vi "Autonomous Independent.vi"() -> ()   [LabVIEW 2012]
doc: "This VI is called when autonomous begins, and will automatically be terminated when autonomous ends. You can carry out timed or sensor driven robot movement independently without needing to return to the caller."
uses:
  Robot Global Data.vi
  <vilib>/Rock Robotics/WPI/RobotDrive/WPI_RobotDriveGetSetRefNum.vi
  <vilib>/Rock Robotics/WPI/Joystick/WPI_JoystickGetSetRefNum.vi
panel:
  out "Current Movement, for debugging":T1 {"Y Joystick Value" scale=1.0..-1.0; "X Joystick Value" scale=-1.0..1.0}
  in  "Array of robot movements":T2(array[cluster]) {"Y Joystick Value" scale=1.0..-1.0; "X Joystick Value" scale=-1.0..1.0}
  # "Be sure to right-click and choose Data Operations>>Make Current Value default if you want to save the array values with the VI"
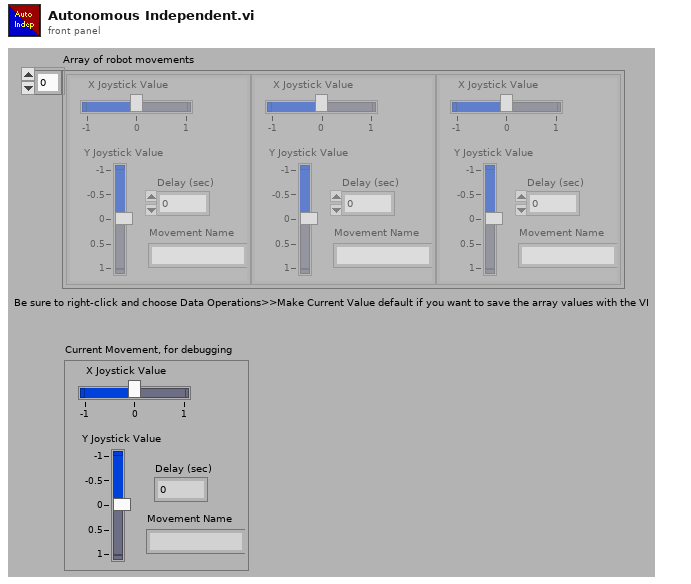
[diagram p1: front panel]
types:
  T1 = cluster{"X Joystick Value":dbl, "Y Joystick Value":dbl, "Delay (sec)":dbl, "Movement Name":string}
  T2 = cluster{"X Joystick Value":dbl, "Y Joystick Value":dbl, "Delay (sec)":dbl, "Movement Name":string}[]
  T3 = typedef "WPI_JoystickDevRef.ctl" = cluster{"Device":T4}
  T4 = typedef "WPI_JoystickDeviceEnum.ctl" = enum16{"USB 1", "USB 2", "USB 3", "USB 4", "Kinect 1", "Kinect 2"}
  T5 = cluster{"axis 1 (x)":dbl, "axis 2 (y)":dbl, "axis 3 (throttle)":dbl, "axis 4":dbl, "axis 5":dbl, "axis 6":dbl}
  T6 = typedef "WPI_RobotDriveDevRef.ctl" = cluster{"DevStatus":errorcluster, "Motors[]":T7[], "Square Inputs":bool, "Max Output":dbl, "Isochronous":bool}
  T7 = typedef "WPI_MotorControlDeviceRef.ctl" = cluster{"DeviceStatus":errorcluster, "Type":enum16{"PWM", "CAN"}, "PWM":cluster{"Digital Module":T8, "PWM Channel":T9, "DeadBand":T10}, "CAN":cluster{"Device Number":u8, "Control Mode":T11, "Semaphore":T12, "Max Vout":dbl}, "Invert":bool, "TransformRef":T13, "InvTransformRef":T13}
  T8 = typedef "FPGA_TypedefDigitalModule.ctl" = enum16{"Digital Module 1", "Digital Module 2"}
  T9 = typedef "FPGA_DIOPWMChannel.ctl" = enum8{"PWM 1", "PWM 2", "PWM 3", "PWM 4", "PWM 5", "PWM 6", "PWM 7", "PWM 8", "PWM 9", "PWM 10", "Invalid"}
  T10 = typedef "WPI_PWMDeadband.ctl" = cluster{"Name":string, "maxPositivePwm":i32, "minPositivePwm":i32, "centerPwm":i32, "maxNegativePwm":i32, "minNegativePwm":i32, "angularRange":u16}
  T11 = typedef "WPI_CANJaguar_ControlMode.ctl" = enum8{"Percent VBus", "Current", "Speed", "Position", "Voltage"}
  T12 = typedef "Semaphore RefNum" = refnum<k1>
  T13 = typedef "WPI_PWMTransform_ConPane.ctl" = refnum<vi>
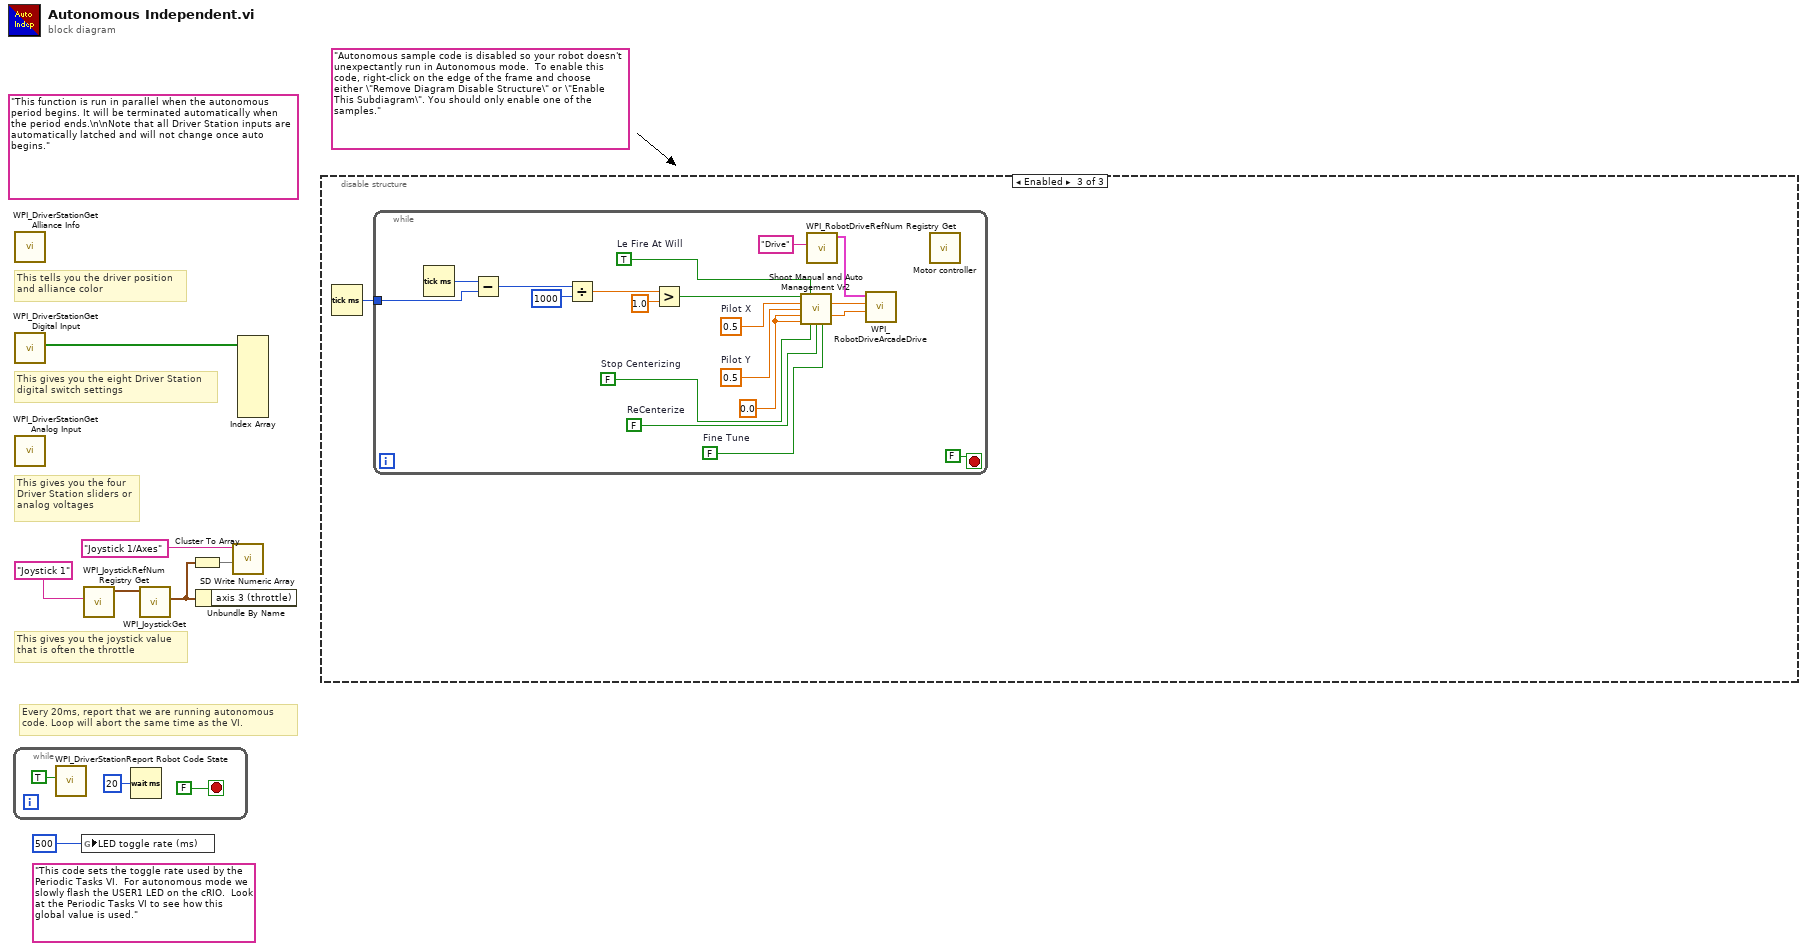
[diagram p0: block diagram]
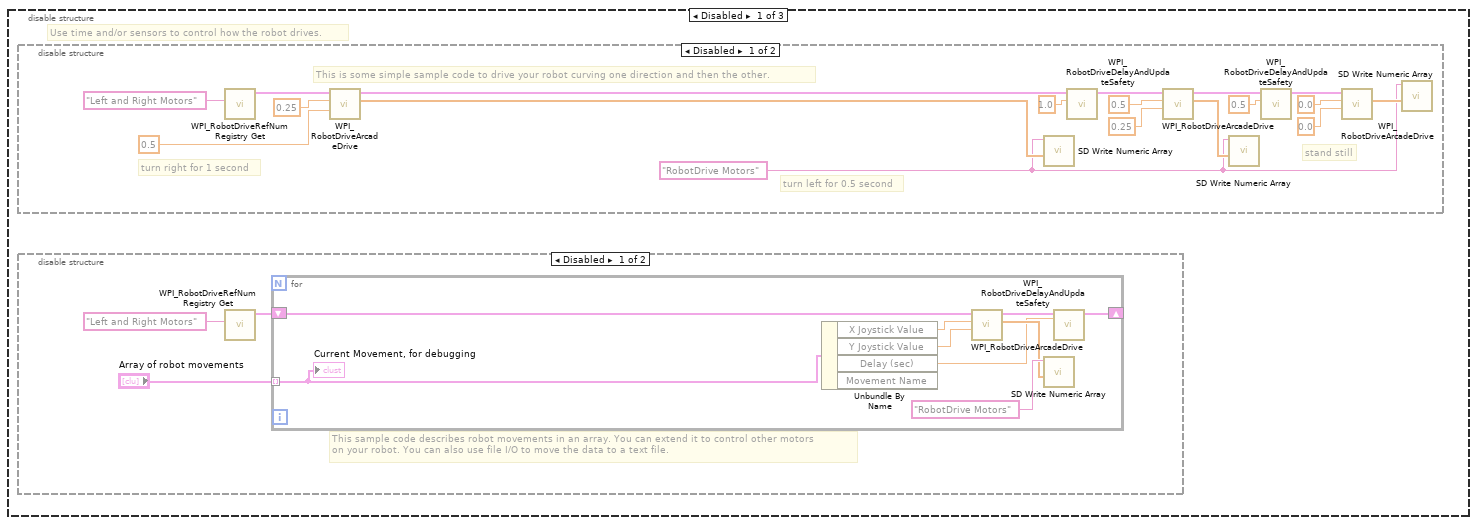
[diagram p2: hidden frame]
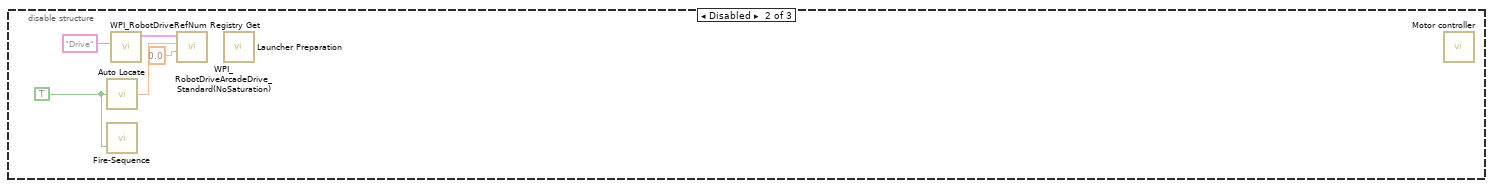
[diagram p5: hidden frame]
diagram:
  (unwired) "This code sets the toggle rate used by the Periodic Tasks VI.  For autonomous mode we slowly flash the USER1 LED on the cRIO.  Look at the Periodic Tasks VI to see how this global value is used."
  (unwired) "Autonomous sample code is disabled so your robot doesn't unexpectantly run in Autonomous mode.  To enable this code, right-click on the edge of the frame and choose either \"Remove Diagram Disable Structure\" or \"Enable This Subdiagram\". You should only enable one of the samples."
  (unwired) "This function is run in parallel when the autonomous period begins. It will be terminated automatically when the period ends.\n\nNote that all Driver Station inputs are automatically latched and will not change once auto begins."
  # "Every 20ms, report that we are running autonomous\ncode. Loop will abort the same time as the VI."
  # "This gives you the joystick value\nthat is often the throttle"
  # "This tells you the driver position\nand alliance color"
  # "This gives you the eight Driver Station\ndigital switch settings"
  # "This gives you the four\nDriver Station sliders or\nanalog voltages"
  n1 = while {
    stop <- FALSE stop-if-true
    n2 = call <vilib>:"WPI_DriverStationReport Robot Code State.vi"("Autonomous"=TRUE) -> ()  [unwired: 10 in, 1 out]
    n3 = Wait (ms)(milliseconds to wait=u32 20) -> ()  [unwired: 1 out]
  }
  n4 = call <vilib>:"WPI_DriverStationGet Alliance Info.vi"() -> ()  [unwired: 12 out]
  n5 = call <vilib>:"WPI_DriverStationGet Digital Input.vi"() -> ("Driver Station Digital Input (1-8)"=w7:bool[])  [unwired: 11 out]
  n6 = call <vilib>:"WPI_DriverStationGet Analog Input.vi"() -> ()  [unwired: 12 out]
  n7 = global write "Robot Global Data.vi" "LED toggle rate (ms)"(u32 500 ("LED ms toggle rate")) -> ()
  n8 = call <vilib>:"WPI_JoystickRefNum Registry Get.vi"("refnum name"="Joystick 1") -> ("JoystickDevRef"=w5:T3)  [unwired: 1 in, 9 out]
  n9 = call <vilib>:"WPI_JoystickGet.vi"("JoystickDevRef"=w5) -> ("Axes"=w2:T5)  [unwired: 1 in, 5 out]
  n10 = Cluster To Array(cluster=w2) -> (array=w3:dbl[])
  n11 = Unbundle By Name(w2) -> ()  [unwired: 1 out]
  n12 = call <vilib>:"SD Write Numeric Array.vi"("Numeric Array"=w3, "Name"="Joystick 1/Axes") -> ()  [unwired: 8 in, 2 out]
  n13 = Index Array(array=w7) -> ()  [unwired: 8 in, 8 out]
  n14 = disable-structure shown="Enabled" {
    frame Disabled {
      # "Use time and/or sensors to control how the robot drives."
      n15 = disable-structure shown="Disabled" {
        frame Disabled {
          w23 = "RobotDrive Motors" ("Name")
          # "This is some simple sample code to drive your robot curving one direction and then the other."
          # "stand still"
          # "turn left for 0.5 second"
          # "turn right for 1 second"
          n16 = call <vilib>:"WPI_RobotDriveRefNum Registry Get.vi"("refnum name"="Left and Right Motors") -> ("RobotDriveDevRef"=w27:T6)  [unwired: 1 in, 9 out]
          n17 = call-poly <vilib>:"WPI_RobotDriveArcadeDrive.vi"("Y axis value"=0.5 ("X axis value"), "X axis value"=0.25, "RobotDriveDevRef"=w27) -> ("Motor Values"=w26:dbl[], "RobotDriveDevRef"=w34:T6)  [unwired: 1 in, 6 out]
          n18 = call <vilib>:"SD Write Numeric Array.vi"("Numeric Array"=w26, "Name"=w23) -> ()  [unwired: 8 in, 2 out]
          n19 = call <vilib>:"WPI_RobotDriveDelayAndUpdateSafety.vi"("Delay (s)"=1.0, "RobotDriveDevRef"=w34) -> ("RobotDriveDevRef 2"=w33:T6)  [unwired: 8 in, 1 out]
          n20 = call-poly <vilib>:"WPI_RobotDriveArcadeDrive.vi"("Y axis value"=0.25 ("X axis value"), "X axis value"=0.5, "RobotDriveDevRef"=w33) -> ("Motor Values"=w25:dbl[], "RobotDriveDevRef"=w32:T6)  [unwired: 1 in, 6 out]
          n21 = call <vilib>:"SD Write Numeric Array.vi"("Numeric Array"=w25, "Name"=w23) -> ()  [unwired: 8 in, 2 out]
          n22 = call <vilib>:"WPI_RobotDriveDelayAndUpdateSafety.vi"("Delay (s)"=0.5, "RobotDriveDevRef"=w32) -> ("RobotDriveDevRef 2"=w31:T6)  [unwired: 8 in, 1 out]
          n23 = call-poly <vilib>:"WPI_RobotDriveArcadeDrive.vi"("Y axis value"=0.0 ("X axis value"), "X axis value"=0.0, "RobotDriveDevRef"=w31) -> ("Motor Values"=w24:dbl[])  [unwired: 1 in, 7 out]
          n24 = call <vilib>:"SD Write Numeric Array.vi"("Numeric Array"=w24, "Name"=w23) -> ()  [unwired: 8 in, 2 out]
        }
        frame Enabled {
        }
      }
      n25 = disable-structure shown="Disabled" {
        frame Disabled {
          # "This sample code describes robot movements in an array. You can extend it to control other motors\non your robot. You can also use file I/O to move the data to a text file."
          n26 = call <vilib>:"WPI_RobotDriveRefNum Registry Get.vi"("refnum name"="Left and Right Motors") -> ("RobotDriveDevRef"=w12:T6)  [unwired: 1 in, 9 out]
          n27 = for {
            shift-right: [w18] -> _
            shift-left: w12 -> [w19]
            tunnel: "Array of robot movements" -> [w14] mode=indexing
            n28 = Unbundle By Name(w14) -> ("X Joystick Value"=w17:dbl, "Y Joystick Value"=w16:dbl, "Delay (sec)"=w15:dbl)  [unwired: 1 out]
            n29 = call-poly <vilib>:"WPI_RobotDriveArcadeDrive.vi"("Y axis value"=w16, "X axis value"=w17, "RobotDriveDevRef"=w19) -> ("Motor Values"=w21:dbl[], "RobotDriveDevRef"=w20:T6)  [unwired: 1 in, 6 out]
            n30 = call <vilib>:"SD Write Numeric Array.vi"("Numeric Array"=w21, "Name"="RobotDrive Motors") -> ()  [unwired: 8 in, 2 out]
            n31 = call <vilib>:"WPI_RobotDriveDelayAndUpdateSafety.vi"("Delay (s)"=w15, "RobotDriveDevRef"=w20) -> ("RobotDriveDevRef 2"=w18:T6)  [unwired: 8 in, 1 out]
            "Current Movement, for debugging" <- w14
          }
        }
        frame Enabled {
        }
      }
    }
    frame Disabled {
      w42 = TRUE
      n32 = call "Auto Locate.vi"("Autonomous?"=w42) -> ("X Drive Arcade"=w41:dbl)
      n33 = call "Fire-Sequence.vi"("La Fire at will?"=w42) -> ()  [unwired: 3 in]
      n34 = call <vilib>:"WPI_RobotDriveRefNum Registry Get.vi"("refnum name"="Drive") -> ("RobotDriveDevRef"=w44:T6)  [unwired: 1 in, 9 out]
      n35 = call <vilib>:"WPI_RobotDriveArcadeDrive_Standard(NoSaturation).vi"("Y axis value"=0.0, "X axis value"=w41, "RobotDriveDevRef"=w44) -> ()  [unwired: 1 in, 8 out]
      n36 = call "Launcher Preparation.vi"() -> ()  [unwired: 5 in]
      n37 = call "Motor controller.vi"() -> ()  [unwired: 12 in]
    }
    frame Enabled {
      n38 = Tick Count (ms)() -> (millisecond timer value=w46:u32)
      n39 = while {
        tunnel: w46 -> [w56]
        stop <- FALSE stop-if-true
        w48 = 0.0 ("Elevation")
        w49 = 0.5  # Pilot Y
        w53 = 0.5  # Pilot X
        w62 = FALSE  # Fine Tune
        w63 = FALSE  # ReCenterize
        w64 = FALSE  # Stop Centerizing
        w65 = TRUE  # Le Fire At Will
        n40 = Tick Count (ms)() -> (millisecond timer value=w57:u32)
        n41 = Subtract(x=w57, y=w56) -> (x-y=w55:u32)
        n42 = Divide(x=w55, y=u32 1000) -> (x/y=w52:dbl)
        n43 = Greater?(x=w52, y=1.0) -> (0:w50:bool)
        n44 = call "Shoot Manual and Auto Management Vr2.vi"("Auto Preparation for Shooting"=w50, "Le Fire At Will"=w65, "Pilot X"=w53, "Pilot Y"=w49, "Elevation"=w48, "Shoot Motors"=w48, "Stop Centerizing"=w64, "ReCenterize"=w63, "Fine Tune"=w62) -> ("X Drive Arcade"=w60:dbl, "Y Drive Arcade"=w59:dbl)  [unwired: 4 in, 1 out]
        n45 = call <vilib>:"WPI_RobotDriveRefNum Registry Get.vi"("refnum name"="Drive") -> ("RobotDriveDevRef"=w58:T6)  [unwired: 9 in, 1 out]
        n46 = call-poly <vilib>:"WPI_RobotDriveArcadeDrive.vi"("Y axis value"=w59, "X axis value"=w60, "RobotDriveDevRef"=w58) -> ()  [unwired: 6 in, 3 out]
        n47 = call "Motor controller.vi"() -> ()  [unwired: 12 in]
      }
    }
  }
